vi "Get Config.vi"(0 "Sequence path":path=path "C:/ModisEdge/Scope/Test Sequence/ModisEdge.ini", 7 "File":string="ModisEdge.ini") -> (1 "Headers Path":path=path "C:/ModisEdge/Scope/Test Sequence/Headers_ModisEdge.ini", 2 "FixtureID":string="MEScope_Fixture1", 3 "StopTestOnFailure":bool=TRUE, 4 "StationID":string="TSNAFT202", 6 "Test Report Path":path=path "C:/Snap-On/ModisEdge_Scope", 8 "DAQ DEVICE NAME":string="Dev5", 10 "WriteTheHeaders":bool, 13 "AlwaysPrint":bool, 14 "UUT_COM":u32=5, 15 "error out":errorcluster)   [LabVIEW 2015]
uses:
  <vilib>/Utility/config.llb/Read Key (Boolean).vi
  <vilib>/Utility/config.llb/Read Key (String).vi
  <vilib>/Utility/config.llb/Read Key (Path).vi
  <vilib>/Utility/config.llb/Read Key (U32).vi
  <vilib>/Utility/config.llb/NI_LVConfig.lvlib
panel:
  out "appended path":path=path "C:/ModisEdge/Scope/Test Sequence/ModisEdge.ini"
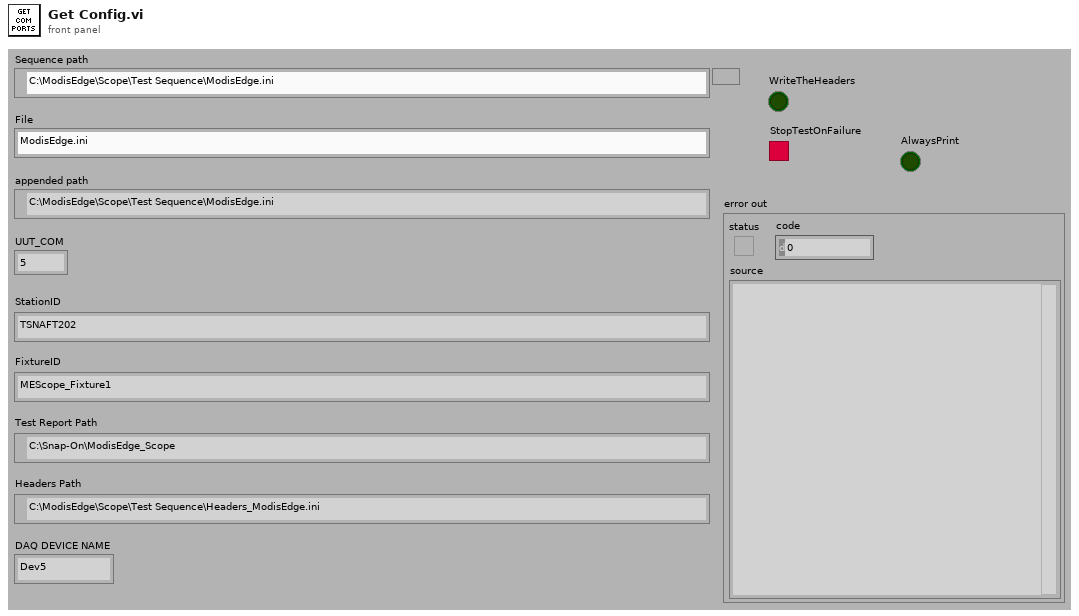
[diagram p1: front panel]
types:
  T1 = typedef "NI_LVConfig.lvlib/Config Data RefNum.ctl" = refnum<k1>
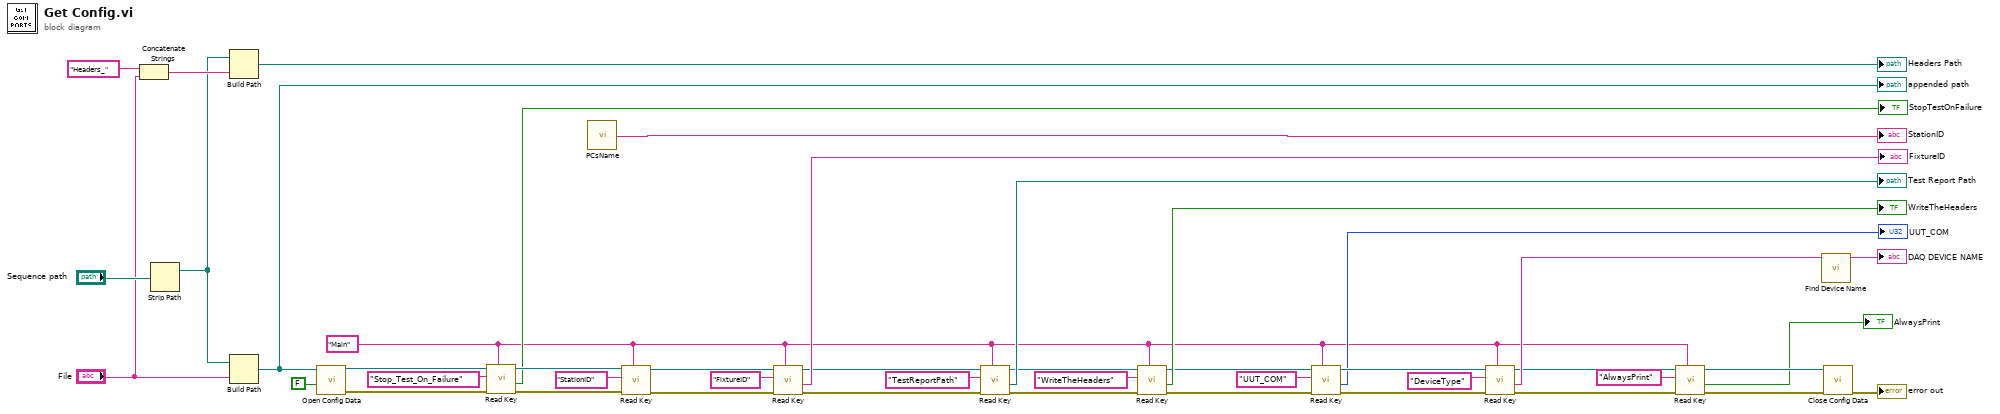
[diagram p0: block diagram]
diagram:
  w3 = "Main" ("section")
  n1 = Concatenate Strings("Headers_", "File") -> (w28:string)
  n2 = Strip Path(path="Sequence path") -> (stripped path=w27:path)  [unwired: 1 out]
  n3 = Build Path(base path=w27, name or relative path=w28) -> (appended path=→"Headers Path":path)
  n4 = Build Path(base path=w27, name or relative path="File") -> (appended path=w25:path)
  "appended path" <- w25
  n5 = call <vilib>:"Open Config Data.vi"("create file if necessary (T)"=FALSE, "configuration file path"=w25) -> ("error out"=w22:errorcluster, "refnum"=w23:T1)  [unwired: 7 in, 1 out]
  n6 = call-poly <vilib>:"Read Key.vi"("section"=w3, "error in (no error)"=w22, "key"="Stop_Test_On_Failure", "refnum"=w23) -> ("error out"=w21:errorcluster, "value"=→"StopTestOnFailure":bool, "refnum out"=w24:T1)  [unwired: 4 in, 1 out]
  n7 = call "PCsName.vi"() -> ("Computer Name"=→"StationID":string)
  n8 = call-poly <vilib>:"Read Key.vi"("section"=w3, "error in (no error)"=w21, "key"="StationID", "refnum"=w24) -> ("error out"=w13:errorcluster, "refnum out"=w9:T1)  [unwired: 4 in, 2 out]
  n9 = call-poly <vilib>:"Read Key.vi"("section"=w3, "error in (no error)"=w13, "key"="FixtureID", "refnum"=w9) -> ("error out"=w12:errorcluster, "value"=→"FixtureID":string, "refnum out"=w10:T1)  [unwired: 4 in, 1 out]
  n10 = call-poly <vilib>:"Read Key.vi"("section"=w3, "error in (no error)"=w12, "key"="TestReportPath", "refnum"=w10) -> ("error out"=w38:errorcluster, "value"=→"Test Report Path":path, "refnum out"=w37:T1)  [unwired: 4 in, 1 out]
  n11 = call-poly <vilib>:"Read Key.vi"("section"=w3, "error in (no error)"=w38, "key"="WriteTheHeaders", "refnum"=w37) -> ("error out"=w32:errorcluster, "value"=→"WriteTheHeaders":bool, "refnum out"=w18:T1)  [unwired: 4 in, 1 out]
  n12 = call-poly <vilib>:"Read Key.vi"("section"=w3, "error in (no error)"=w32, "key"="UUT_COM", "refnum"=w18) -> ("error out"=w19:errorcluster, "value"=→"UUT_COM":u32, "refnum out"=w17:T1)  [unwired: 4 in, 1 out]
  n13 = call-poly <vilib>:"Read Key.vi"("section"=w3, "error in (no error)"=w19, "key"="DeviceType", "refnum"=w17) -> ("error out"=w7:errorcluster, "value"=w31:string, "refnum out"=w6:T1)  [unwired: 4 in, 1 out]
  n14 = call-poly <vilib>:"Read Key.vi"("section"=w3, "error in (no error)"=w7, "key"="AlwaysPrint", "refnum"=w6) -> ("error out"=w4:errorcluster, "value"=→"AlwaysPrint":bool, "refnum out"=w5:T1)  [unwired: 4 in, 1 out]
  n15 = call "Find Device Name.vi"("Device Type"=w31) -> ("Device Name"=→"DAQ DEVICE NAME":string)  [unwired: 10 in]
  n16 = call <vilib>:"Close Config Data.vi"("error in (no error)"=w4, "refnum"=w5) -> ("error out"=→"error out":errorcluster)  [unwired: 8 in, 1 out]
